vi "Teleop.vi"(10 "Match Info":T1={"Autonomous Elapsed Seconds"=0.0, "TeleOp Elapsed Seconds"=0.0, "Disabled Elapsed Seconds"=0.0, "Visited Autonomous"=FALSE, "Visited TeleOp"=FALSE, "Visited Disabled"=FALSE, "Autonomous Settings"={"Autonomous Style"=enum."Independent", "VI Refnum"=refnum}}, 11 "Call Context":T2) -> ()   [LabVIEW 2013]
doc: "This VI is called for each TeleOp packet received from the DS where the robot is not disabled. It is often used to read from the joysticks and update I/O or to update setpoints for timed control loops. It should complete and return within 20 milliseconds or it may miss DS packets."
uses:
  <vilib>/Rock Robotics/WPI/DriverStation/WPI_DriverStationDerivedRobotMode.ctl
  <vilib>/Rock Robotics/WPI/DriverStation/WPI_DriverStationMatch Info.ctl
  Robot Global Data.vi
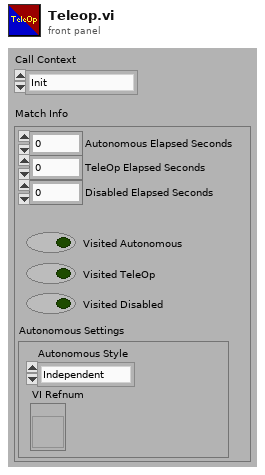
[diagram p1: front panel]
types:
  T1 = typedef "WPI_DriverStationMatch Info.ctl" = cluster{"Autonomous Elapsed Seconds":dbl, "TeleOp Elapsed Seconds":dbl, "Disabled Elapsed Seconds":dbl, "Visited Autonomous":bool, "Visited TeleOp":bool, "Visited Disabled":bool, "Autonomous Settings":cluster{"Autonomous Style":enum16{"Iterative", "Independent"}, "VI Refnum":refnum<vi>}}
  T2 = typedef "WPI_DriverStationDerivedRobotMode.ctl" = enum16{"Init", "Execute", "Stop"}
  T3 = typedef "Joystick Data.ctl" = cluster{"Joystick 1 Axes":cluster{"x":dbl, "y":dbl, "z":dbl, "Throttle":dbl}, "Joystick 2 Axes":cluster{"x":dbl, "y":dbl, "z":dbl, "Throttle":dbl}, "Buttons":cluster{"Shoot":bool, "Low Gear":bool, "High Gear":bool, "Grab out":bool, "Catch":bool, "Grab in":bool, "Pass":bool, "Manual Arm Out":bool, "Manual Arm In":bool, "Manual Shoot":bool, "Manual Air Compressor On":bool, "Manual Air Compressor Off":bool, "Manual Fingers Open":bool, "Manual Fingers Close":bool, "Manual Rollers In":bool, "Manual Rollers Out":bool, "Reset":bool, "Kachig Left":bool, "Kachig Right":bool, "Truss Shot":bool}}
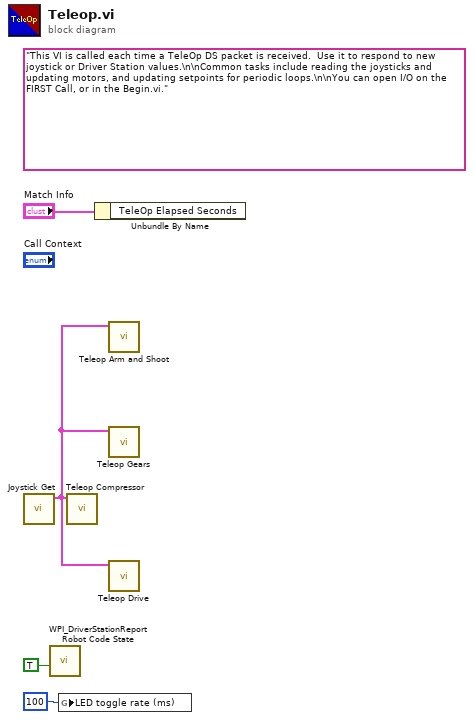
[diagram p0: block diagram]
diagram:
  (unwired) "This VI is called each time a TeleOp DS packet is received.  Use it to respond to new joystick or Driver Station values.\n\nCommon tasks include reading the joysticks and updating motors, and updating setpoints for periodic loops.\n\nYou can open I/O on the FIRST Call, or in the Begin.vi."
  n1 = call "Joystick Get.vi"() -> ("Mapped Data"=w1:T3)  [unwired: 9 in, 2 out]
  n2 = call <vilib>:"WPI_DriverStationReport Robot Code State.vi"("TeleOp"=TRUE ("Autonomous")) -> ()  [unwired: 10 in, 1 out]
  n3 = global write "Robot Global Data.vi" "LED toggle rate (ms)"(u32 100 ("LED ms toggle rate")) -> ()
  n4 = call "Teleop Compressor.vi"("Joystick Data"=w1) -> ()  [unwired: 11 in]
  n5 = Unbundle By Name("Match Info") -> ()  [unwired: 1 out]
  n6 = call "Teleop Arm and Shoot.vi"("Joystick Data"=w1) -> ()  [unwired: 11 in]
  n7 = call "Teleop Gears.vi"("Joystick Data"=w1) -> ()  [unwired: 11 in]
  n8 = call "Teleop Drive.vi"("Joystick Data"=w1) -> ()  [unwired: 11 in]
